vi "Close.vi"(8 "Error in":errorcluster, 11 "VISA resource name":refnum<visa-resource-name>) -> (0 "Error out":errorcluster)   [LabVIEW 2020, in "plugin_flodx_pressure.lvlib" / "mock_driver.lvlib"]
doc: "Simulates closing the connection."
uses:
  mock_driver.lvlib
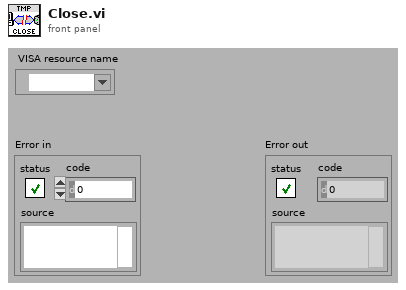
[diagram p1: front panel]
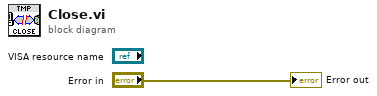
[diagram p0: block diagram]
diagram:
  "Error out" <- "Error in"
